vi "RotateVector.vi"(0 "CirculateSkill in":refnum<class "CirculateSkill.lvclass">, 5 "Vector in":dbl[](array[numeric]), 7 "rotationAngle":dbl, 9 "Clockwise?":bool, 11 "error in (no error)":errorcluster) -> (4 "CirculateSkill out":refnum<class "CirculateSkill.lvclass">, 6 "Vector out":dbl[](array[numeric]), 15 "error out":errorcluster)   [LabVIEW 2023, in "CirculateSkill.lvclass"]
uses:
  CirculateSkill.lvclass
  <vilib>/Analysis/coordinate.llb/2D Cartesian Coordinate Rotation (Scalar).vi
  CirculateSkill.lvclass/CirculateSkill.ctl
  <vilib>/Analysis/NI_AALPro.lvlib
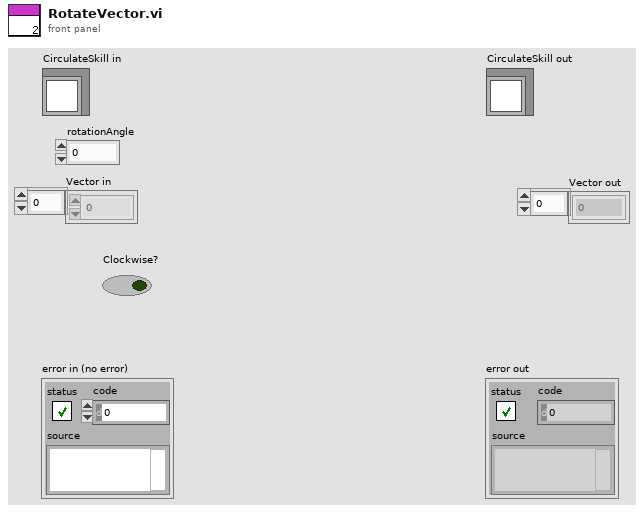
[diagram p1: front panel]
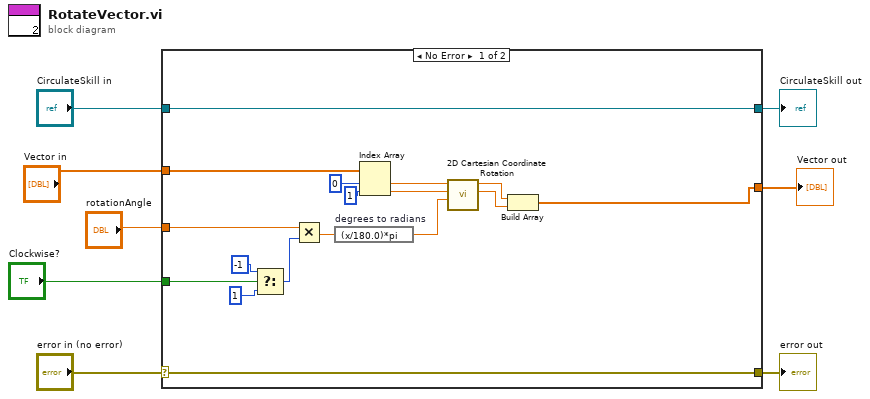
[diagram p0: block diagram]
diagram:
  n1 = case shown="No Error" "error in (no error)" {
    selector: "error in (no error)" -> [w24 w28]
    tunnel: [w24 w28] -> w7
    tunnel: [w25 w27] -> w5
    tunnel: "CirculateSkill in" -> [w25 w27]
    tunnel: "Vector in" -> [w12 w26]
    tunnel: "Clockwise?" -> [w9 _]
    tunnel: [w10 w26] -> w2
    tunnel: "rotationAngle" -> [w11 _]
    frame No Error {
      n2 = Select(t=-1, s=w9, f=1) -> (s? t:f=w21:i32)
      n3 = Multiply(x=w11, y=w21) -> (x*y=w18:dbl)
      n4 = expression code="(x/180.0)*pi" "degrees to radians"(w18) -> (w17:dbl)
      n5 = Index Array(array=w12, index #1=0 ("index"), index #2=1 ("index")) -> (element #1=w14:dbl, element #2=w13:dbl)
      n6 = call-poly <vilib>:"2D Cartesian Coordinate Rotation.vi"("theta"=w17, "y"=w13, "x"=w14) -> ("y out"=w15:dbl, "x out"=w16:dbl)  [unwired: 6 in, 1 out]
      n7 = Build Array(w16, w15) -> (w10:dbl[])
    }
    frame Error {
    }
  }
  "error out" <- w7
  "CirculateSkill out" <- w5
  "Vector out" <- w2
